vi "svacg_LimitTest Check resampled Length.vi"(4 "Protection limits":T1={"Max oversampling ratio"=1024.0, "Max # output samples"=2097150}, 8 "error in":errorcluster, 9 "x0 in":dbl=1.0 format="%.2p", 10 "dx in":dbl format="%.2p", 11 "Specification Cluster":cluster{"X":dbl[], "Y":dbl[]}[](array[cluster]) {"Y" format="%.2p"; "X" format="%.2p"}) -> (0 "error out":errorcluster, 1 "x0 out":dbl=1.0 format="%.2p", 2 "dx out":dbl format="%.2p", 3 "Specification Cluster out":cluster{"X":dbl[], "Y":dbl[]}[](array[cluster]) {"Y" format="%.2p"; "X" format="%.2p"})   [LabVIEW 2017]
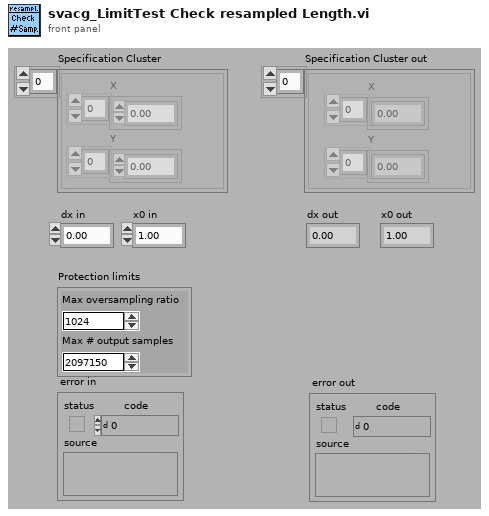
[diagram p1: front panel]
types:
  T1 = cluster{"Max oversampling ratio":dbl, "Max # output samples":i32}
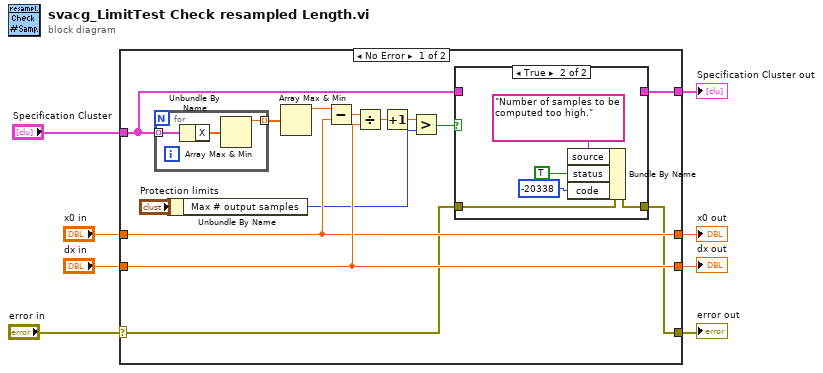
[diagram p0: block diagram]
diagram:
  n1 = case shown="No Error" "error in" {
    selector: "error in" -> [w12 w35]
    tunnel: [w11 w35] -> w7
    tunnel: "Specification Cluster" -> [w10 _]
    tunnel: "x0 in" -> [w16 w34]
    tunnel: "dx in" -> [w17 w33]
    tunnel: [w17 w33] -> w3
    tunnel: [w16 w34] -> w2
    tunnel: [w9 _] -> w1
    frame No Error {
      n2 = for {
        tunnel: w10 -> [w32] mode=indexing
        tunnel: [w30] -> w22 mode=indexing
        n3 = Unbundle By Name(w32) -> ("X"=w31:dbl[])
        n4 = Array Max & Min(array=w31) -> (max value=w30:dbl)  [unwired: 3 out]
      }
      n5 = Unbundle By Name("Protection limits") -> ("Max # output samples"=w14:i32)
      n6 = Array Max & Min(array=w22) -> (max value=w21:dbl)  [unwired: 3 out]
      n7 = Subtract(x=w21, y=w16) -> (x-y=w20:dbl)
      n8 = Divide(x=w20, y=w17) -> (x/y=w19:dbl)
      n9 = Increment(x=w19) -> (x+1=w18:dbl)
      n10 = Greater?(x=w18, y=w14) -> (0:w13:bool)
      n11 = case shown="True" w13 {
        tunnel: w12 -> [w24 w27]
        tunnel: [w24 w26] -> w11
        tunnel: [w23 _] -> w9
        tunnel: w10 -> [w23 _]
        frame False {
        }
        frame True {
          n12 = Bundle By Name(cluster=w27, "source"="Number of samples to be computed too high.", "status"=TRUE, "code"=-20338) -> (w26:errorcluster)
        }
      }
    }
    frame Error {
    }
  }
  "error out" <- w7
  "Specification Cluster out" <- w1
  "dx out" <- w3
  "x0 out" <- w2
